vi "DataSimGen.vi"(0 "multiplicateur":dbl, 5 "Données":enum16{"crv 1", "crv 2", "crv 3", "crv 123"}(ring), 11 "error in (no error)":errorcluster, 12 "Gen Mult":bool, 13 "IndicePoint":i32) -> (2 "Outputs":dbl[](array[numeric]), 4 "multiplicateur out":dbl, 6 "Output":dbl format="%.4e", 15 "error out":errorcluster)   [LabVIEW 2019]
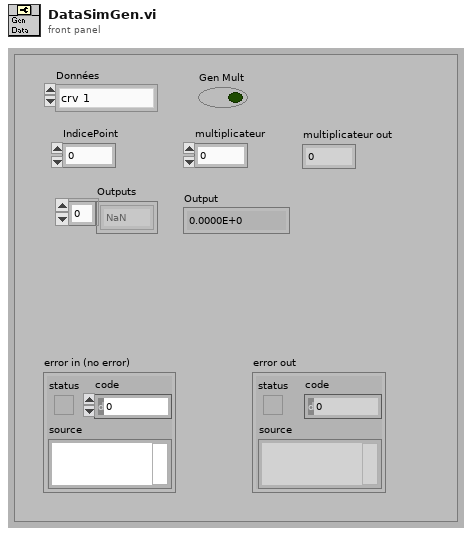
[diagram p1: front panel]
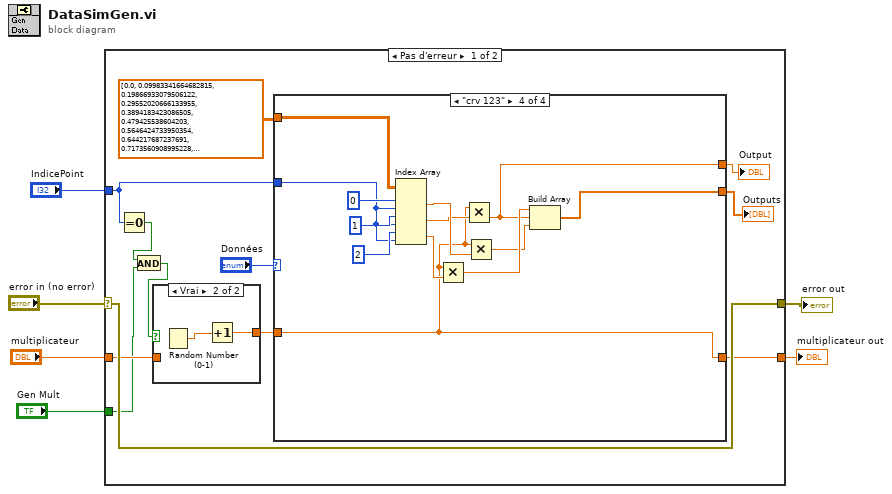
[diagram p0: block diagram]
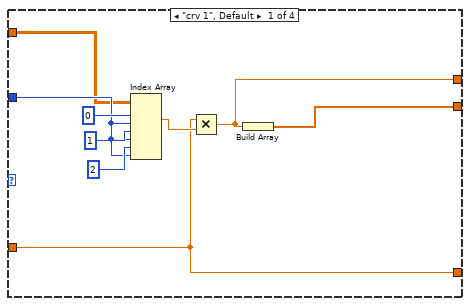
[diagram p3: hidden frame]
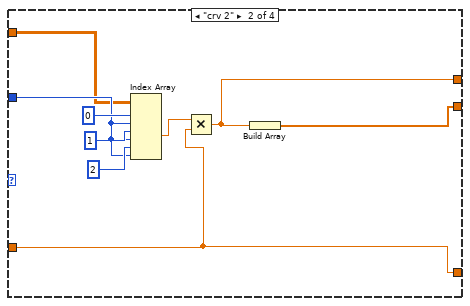
[diagram p4: hidden frame]
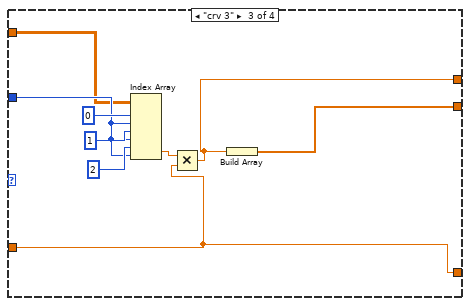
[diagram p5: hidden frame]
diagram:
  n1 = case shown="Pas d'erreur" "error in (no error)" {
    selector: "error in (no error)" -> [w17 w63]
    tunnel: [w17 w63] -> w5
    tunnel: "multiplicateur" -> [w13 w62]
    tunnel: [w12 w62] -> w3
    tunnel: "IndicePoint" -> [w10 _]
    tunnel: "Gen Mult" -> [w8 _]
    frame No Error {
      n2 = Equal To 0?(x=w10) -> (x = 0?=w9:bool)
      n3 = And(x=w9, y=w8) -> (x .and. y?=w7:bool)
      n4 = case shown="Vrai" w7 {
        tunnel: [w19 w20] -> w14
        tunnel: w13 -> [w19 _]
        frame False {
        }
        frame True {
          n5 = Random Number (0-1)() -> (number: 0 to 1=w21:dbl)
          n6 = Increment(x=w21) -> (x+1=w20:dbl)
        }
      }
      n7 = case shown="\"crv 123\"" "Données" {
        tunnel: w10 -> [w27 w36 w45 w56]
        tunnel: [w26 w35 w44 w55] -> w15
        tunnel: [w24 w33 w42 w51] -> w16
        tunnel: w14 -> [w23 w32 w41 w50]
        tunnel: [w23 w32 w41 w50] -> w12
        tunnel: dbl[][] [[0.0, 0.09983341664682815, 0.19866933079506122, 0.29552020666133955, 0.3894183423086505, 0.479425538604203, 0.5646424733950354, 0.644217687237691, 0.7173560908995228, 0.7833269096274834, 0.8414709848078965, 0.8912073600614354, 0.9320390859672263, 0.963558185417193, 0.9854497299884601, 0.9974949866040544, 0.9995736030415051, 0.9916648104524686, 0.9738476308781951, 0.9463000876874145, 0.9092974268256817, 0.8632093666488737, 0.8084964038195901, 0.7457052121767203, 0.675463180551151, 0.5984721441039564, 0.5155013718214642, 0.4273798802338298, 0.3349881501559051, 0.23924932921398243, 0.1411200080598672, 0.04158066243329049, -0.058374143427580086, -0.1577456941432482, -0.2555411020268312, -0.35078322768961984, -0.44252044329485246, -0.5298361409084934, -0.6118578909427189, -0.6877661591839738, -0.7568024953079282, -0.8182771110644103, -0.8715757724135882, -0.9161659367494549, -0.951602073889516, -0.977530117665097, -0.9936910036334644, -0.9999232575641008, -0.9961646088358407, -0.9824526126243325, -0.9589242746631385, -0.9258146823277325, -0.8834546557201531, -0.8322674422239013, -0.7727644875559871, -0.7055403255703919, -0.6312666378723216, -0.5506855425976376, -0.46460217941375737, -0.373876664830236, -0.27941549819892586, -0.18216250427209588, -0.0830894028174964, 0.016813900484349713, 0.11654920485049364, 0.21511998808781552, 0.31154136351337786, 0.4048499206165983, 0.49411335113860816, 0.5784397643882001, 0.6569865987187891, 0.7289690401258759, 0.7936678638491531, 0.8504366206285644, 0.8987080958116269, 0.9379999767747389, 0.9679196720314863, 0.9881682338770004, 0.998543345374605, 0.998941341839772, 0.9893582466233818, 0.9698898108450863, 0.9407305566797731, 0.9021718337562933, 0.8545989080882804, 0.7984871126234903, 0.7343970978741133, 0.6629692300821833, 0.5849171928917617, 0.5010208564578846, 0.4121184852417566, 0.3190983623493521, 0.22288991410024764, 0.1244544235070617, 0.024775425453357765, -0.0751511204618093, -0.17432678122297965, -0.27176062641094245, -0.36647912925192844, -0.45753589377532133], [1.0, 0.9950041652780258, 0.9800665778412416, 0.955336489125606, 0.9210609940028851, 0.8775825618903728, 0.8253356149096783, 0.7648421872844885, 0.6967067093471654, 0.6216099682706644, 0.5403023058681398, 0.4535961214255773, 0.3623577544766736, 0.26749882862458735, 0.16996714290024104, 0.0707372016677029, -0.029199522301288815, -0.12884449429552464, -0.2272020946930871, -0.32328956686350335, -0.4161468365471424, -0.5048461045998576, -0.5885011172553458, -0.6662760212798241, -0.7373937155412454, -0.8011436155469337, -0.8568887533689473, -0.9040721420170612, -0.9422223406686581, -0.9709581651495905, -0.9899924966004454, -0.9991351502732795, -0.9982947757947531, -0.9874797699088649, -0.9667981925794611, -0.9364566872907963, -0.896758416334147, -0.848100031710408, -0.7909677119144168, -0.7259323042001402, -0.6536436208636119, -0.5748239465332692, -0.4902608213406994, -0.40079917207997545, -0.30733286997841935, -0.2107957994307797, -0.11215252693505487, -0.01238866346289056, 0.0874989834394464, 0.18651236942257576, 0.28366218546322625, 0.37797774271298024, 0.4685166713003771, 0.5543743361791608, 0.6346928759426347, 0.70866977429126, 0.7755658785102496, 0.8347127848391598, 0.8855195169413189, 0.9274784307440359, 0.960170286650366, 0.9832684384425845, 0.9965420970232175, 0.9998586363834151, 0.9931849187581926, 0.9765876257280235, 0.9502325919585296, 0.9143831482353194, 0.8693974903498253, 0.8157251001253568, 0.7539022543433046, 0.6845466664428066, 0.6083513145322546, 0.5260775173811053, 0.43854732757439036, 0.3466353178350258, 0.2512598425822557, 0.15337386203786435, 0.05395542056264975, -0.04600212563953695, -0.14550003380861354, -0.2435441537357911, -0.3391548609838345, -0.4313768449706208, -0.5192886541166856, -0.6020119026848236, -0.6787200473200125, -0.7486466455973987, -0.811093014061656, -0.8654352092411123, -0.9111302618846769, -0.9477216021311119, -0.9748436214041636, -0.9922253254526034, -0.9996930420352065, -0.9971721561963784, -0.984687855794127, -0.9623648798313102, -0.9304262721047533, -0.8891911526253609], [5e-05, 5.525854590378239e-05, 6.10701379080085e-05, 6.749294037880016e-05, 7.459123488206351e-05, 8.24360635350064e-05, 9.110594001952544e-05, 0.00010068763537352383, 0.0001112770464246234, 0.0001229801555578475, 0.00013591409142295224, 0.00015020830119732168, 0.00016600584613682737, 0.0001834648333809622, 0.00020275999834223373, 0.00022408445351690322, 0.00024765162121975575, 0.00027369736958636, 0.00030248237322064733, 0.0003342947221139634, 0.00036945280494653254, 0.0004083084956283826, 0.0004512506749717061, 0.0004987091227407359, 0.0005511588190320801, 0.0006091246980351737, 0.0006731869017500845, 0.0007439865862436418, 0.0008222323385548524, 0.0009087072684721531, 0.0010042768461593834, 0.001109897564072082, 0.0012266265098554677, 0.001355631946032894, 0.0014982050023698505, 0.0016557725979346157, 0.0018299117221838993, 0.00202236521800337, 0.0022350592246650407, 0.0024701224552765083, 0.0027299075016572116, 0.0030170143798680976, 0.0033343165520462576, 0.0036849896849797895, 0.004072543433248407, 0.00450085656502609, 0.004974215782096689, 0.005497358622606177, 0.0060755208759367425, 0.006714488984246776, 0.00742065795512883, 0.008201095364995085, 0.009063612093757561, 0.010016840498739583, 0.011070320810209358, 0.012234596613211019, 0.013521320371307627, 0.014943370048353015, 0.016514977995482433, 0.018251873393266446, 0.020171439674636756, 0.02229288850412584, 0.024637452054662817, 0.02722859550629645, 0.03009225189360411, 0.03325708165221809, 0.036754759462098635, 0.04062029125837716, 0.044892364582520876, 0.049613735780251314, 0.05483165792142292, 0.060598353724628816, 0.0669715382197209, 0.07401499637922725, 0.08179922149979635, 0.09040212072280315, 0.09990979475520587, 0.11041739959436045, 0.12203009888122492, 0.1348641164134255, 0.14904789935208643, 0.164723403764192, 0.18204751536661762, 0.20119361969111565, 0.22235333738499288, 0.2457384420149567, 0.2715829795681489, 0.3001456108630509, 0.3317122003138945, 0.36659867695779974, 0.4051541963787692, 0.4477646351741254, 0.49485645293719543, 0.5469009604082595, 0.6044190365108494, 0.6679863414830937, 0.7382390782788634, 0.815880359900771, 0.9016872463914262, 0.9965185219115148]] ("tableau ajouté") -> [w22 w31 w40 w49]
        frame "crv 1", Default {
          n8 = Index Array(array=w22, index (row) #1=0 ("indice (ligne)"), index (col) #1=w27, index (row) #2=1 ("indice (ligne)"), index (col) #2=w27, index (row) #3=2 ("indice (ligne)"), index (col) #3=w27) -> (element #1=w25:dbl)  [unwired: 2 out]
          n9 = Multiply(x=w23, y=w25) -> (x*y=w24:dbl)
          n10 = Build Array(w24) -> (w26:dbl[])
        }
        frame "crv 2" {
          n11 = Index Array(array=w31, index (row) #1=0 ("indice (ligne)"), index (col) #1=w36, index (row) #2=1 ("indice (ligne)"), index (col) #2=w36, index (row) #3=2 ("indice (ligne)"), index (col) #3=w36) -> (element #2=w34:dbl)  [unwired: 2 out]
          n12 = Multiply(x=w34, y=w32) -> (x*y=w33:dbl)
          n13 = Build Array(w33) -> (w35:dbl[])
        }
        frame "crv 3" {
          n14 = Index Array(array=w40, index (row) #1=0 ("indice (ligne)"), index (col) #1=w45, index (row) #2=1 ("indice (ligne)"), index (col) #2=w45, index (row) #3=2 ("indice (ligne)"), index (col) #3=w45) -> (element #3=w43:dbl)  [unwired: 2 out]
          n15 = Multiply(x=w43, y=w41) -> (x*y=w42:dbl)
          n16 = Build Array(w42) -> (w44:dbl[])
        }
        frame "crv 123" {
          n17 = Index Array(array=w49, index (row) #1=0 ("indice (ligne)"), index (col) #1=w56, index (row) #2=1 ("indice (ligne)"), index (col) #2=w56, index (row) #3=2 ("indice (ligne)"), index (col) #3=w56) -> (element #1=w61:dbl, element #2=w54:dbl, element #3=w60:dbl)
          n18 = Multiply(x=w50, y=w60) -> (x*y=w53:dbl)
          n19 = Multiply(x=w50, y=w54) -> (x*y=w51:dbl)
          n20 = Multiply(x=w50, y=w61) -> (x*y=w52:dbl)
          n21 = Build Array(w53, w51, w52) -> (w55:dbl[])
        }
      }
      "Outputs" <- w15
      "Output" <- w16
    }
    frame Error {
    }
  }
  "error out" <- w5
  "multiplicateur out" <- w3
